vi "test Finalize Validation.vi"(8 "error in (no error)":errorcluster, 11 "TestCase in":refnum<class "Routing and Faulting Validation Unit Tests.lvclass">) -> (0 "error out":errorcluster, 3 "TestCase out":refnum<class "Routing and Faulting Validation Unit Tests.lvclass">)   [LabVIEW 2020, in "Routing and Faulting Validation Unit Tests.lvclass"]
uses:
  Routing and Faulting Validation Unit Tests.lvclass
  Routing and Faulting Validation Unit Tests.lvclass/Routing and Faulting Validation Unit Tests.ctl
  NationalInstruments.VeriStand.SystemStorage
  Constants/Scripting Constants.vi
  <vilib>/addons/_JKI Toolkits/VI Tester/TestCase.llb/TestCase.lvclass
  <vilib>/NI VeriStand/Custom Device API/Custom Device API.lvlib
  Routing and Faulting Scripting.lvlib
  C:/Program Files (x86)/National Instruments/LabVIEW 2020/vi.lib/addons/_JKI Toolkits/VI Tester/TestCase.llb/TestCase.lvclass
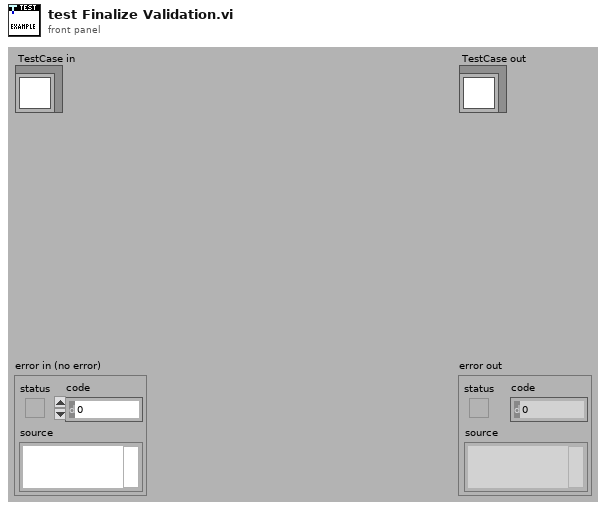
[diagram p1: front panel]
types:
  T1 = typedef "Custom Device API.lvlib/Custom Device Item Ref.ctl" = u64
  T2 = typedef "Routing and Faulting Scripting.lvlib/Validation Information.ctl" = cluster{"Missing Modules":variant, "Module Connection Map":variant, "Unused Modules":variant}
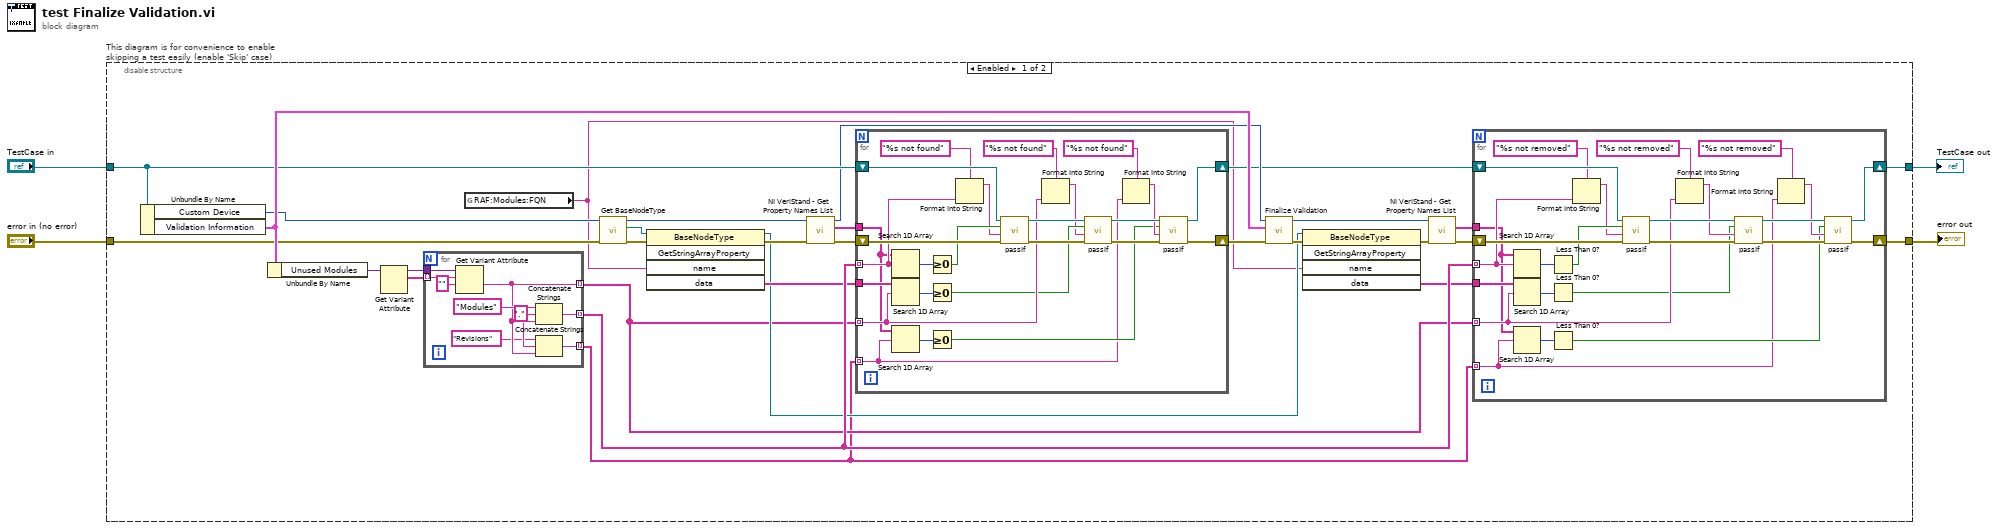
[diagram p0: block diagram]
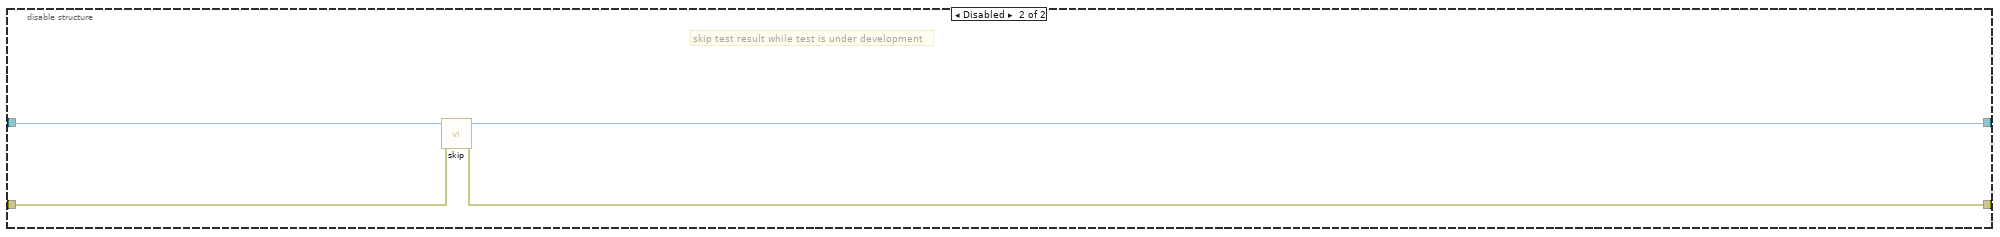
[diagram p2: hidden frame]
diagram:
  n1 = disable-structure "This diagram is for convenience to enable skipping a test easily (enable 'Skip' case)" shown="Enabled" {
    disable-tunnel: "TestCase in" -> [w29 w97]
    disable-tunnel: [w24 w95] -> w1
    disable-tunnel: [w23 w96] -> w3
    disable-tunnel: "error in (no error)" -> [w18 w94]
    frame Enabled {
      n2 = Unbundle By Name(w29) -> ("Custom Device"=w17:T1, "Validation Information"=w33:T2)
      n3 = Unbundle By Name(w33) -> ("Unused Modules"=w32:variant)
      n4 = Get Variant Attribute(Variant=w32) -> (duplicate Variant=w31:variant, names=w30:string[])  [unwired: 3 in, 2 out]
      n5 = for {
        tunnel: w31 -> [w93]
        tunnel: w30 -> [w92] mode=indexing
        tunnel: [w90] -> w19 mode=indexing
        tunnel: [w88] -> w6 mode=indexing
        tunnel: [w85] -> w5 mode=indexing
        w87 = "." ("string")
        n6 = Get Variant Attribute(Variant=w93, name=w92, default value (empty Variant)="") -> (value=w88:string)  [unwired: 1 in, 3 out]
        n7 = Concatenate Strings("Modules" ("string"), w87, w88) -> (w90:string)
        n8 = Concatenate Strings("Revisions" ("string"), w87, w88) -> (w85:string)
      }
      n9 = global read "Scripting Constants.vi" "RAF:Modules:FQN"() -> (w8:string)
      n10 = call "Get BaseNodeType.vi"("error in"=w18, "item in"=w17) -> ("error out"=w15:errorcluster, "BaseNodeType"=w14:refnum<k24>, "item out"=w16:T1)  [unwired: 7 in]
      n11 = invoke class="BaseNodeType" method="GetStringArrayProperty"(reference=w14, error in=w15, "name"=w8) -> (reference out=w9:refnum<k24>, error out=w13:errorcluster, "data"=w12:string[])  [unwired: 2 in, 2 out]
      n12 = call <vilib>:"NI VeriStand - Get Property Names List.vi"("error in (no error)"=w13, "Item Ref in"=w16) -> ("error out"=w28:errorcluster, "Property Names"=w27:string[], "Item Ref out"=w25:T1)  [unwired: 7 in]
      n13 = for {
        shift-right: [w66] -> w22
        shift-left: w29 -> [w81]
        shift-right: [w65] -> w26
        shift-left: w28 -> [w84]
        tunnel: w27 -> [w61]
        tunnel: w19 -> [w78] mode=indexing
        tunnel: w6 -> [w74] mode=indexing
        tunnel: w12 -> [w69]
        tunnel: w5 -> [w60] mode=indexing
        n14 = Search 1D Array(1D array=w61, element=w78) -> (index of element=w83:i32)  [unwired: 1 in]
        n15 = Search 1D Array(1D array=w69, element=w74) -> (index of element=w73:i32)  [unwired: 1 in]
        n16 = Search 1D Array(1D array=w61, element=w60) -> (index of element=w70:i32)  [unwired: 1 in]
        n17 = Greater Or Equal To 0?(x=w83) -> (x >= 0?=w82:bool)
        n18 = Greater Or Equal To 0?(x=w73) -> (x >= 0?=w72:bool)
        n19 = Greater Or Equal To 0?(x=w70) -> (x >= 0?=w62:bool)
        n20 = Format Into String(format string="%s not found" ("message (\"\")"), w78) -> (resulting string=w79:string)  [unwired: 2 in, 1 out]
        n21 = call-dynamic "passIf.vi"("error in (no error)"=w84, "message (\"\")"=w79, "pass"=w82, "TestCase in"=w81) -> ("error out"=w77:errorcluster, "TestCase out"=w76:refnum<class "Routing and Faulting Validation Unit Tests.lvclass">)  [unwired: 6 in]
        n22 = Format Into String(format string="%s not found" ("message (\"\")"), w74) -> (resulting string=w71:string)  [unwired: 2 in, 1 out]
        n23 = call-dynamic "passIf.vi"("error in (no error)"=w77, "message (\"\")"=w71, "pass"=w72, "TestCase in"=w76) -> ("error out"=w68:errorcluster, "TestCase out"=w67:refnum<class "Routing and Faulting Validation Unit Tests.lvclass">)  [unwired: 6 in]
        n24 = Format Into String(format string="%s not found" ("message (\"\")"), w60) -> (resulting string=w63:string)  [unwired: 2 in, 1 out]
        n25 = call-dynamic "passIf.vi"("error in (no error)"=w68, "message (\"\")"=w63, "pass"=w62, "TestCase in"=w67) -> ("error out"=w65:errorcluster, "TestCase out"=w66:refnum<class "Routing and Faulting Validation Unit Tests.lvclass">)  [unwired: 6 in]
      }
      n26 = call "Finalize Validation.vi"("error in"=w26, "validation information"=w33, "routing and faulting in"=w25) -> ("error out"=w10:errorcluster, "routing and faulting out"=w34:T1)  [unwired: 7 in]
      n27 = invoke class="BaseNodeType" method="GetStringArrayProperty"(reference=w9, error in=w10, "name"=w8) -> (error out=w11:errorcluster, "data"=w7:string[])  [unwired: 2 in, 3 out]
      n28 = call <vilib>:"NI VeriStand - Get Property Names List.vi"("error in (no error)"=w11, "Item Ref in"=w34) -> ("error out"=w21:errorcluster, "Property Names"=w20:string[])  [unwired: 7 in, 1 out]
      n29 = for {
        shift-right: [w39] -> w24
        shift-left: w22 -> [w56]
        shift-right: [w38] -> w23
        shift-left: w21 -> [w59]
        tunnel: w20 -> [w44]
        tunnel: w19 -> [w53] mode=indexing
        tunnel: w7 -> [w48]
        tunnel: w6 -> [w47] mode=indexing
        tunnel: w5 -> [w35] mode=indexing
        n30 = Search 1D Array(1D array=w44, element=w53) -> (index of element=w58:i32)  [unwired: 1 in]
        n31 = Search 1D Array(1D array=w48, element=w47) -> (index of element=w46:i32)  [unwired: 1 in]
        n32 = Search 1D Array(1D array=w44, element=w35) -> (index of element=w43:i32)  [unwired: 1 in]
        n33 = Less Than 0?(x=w58) -> (x < 0?=w57:bool)
        n34 = Less Than 0?(x=w46) -> (x < 0?=w45:bool)
        n35 = Less Than 0?(x=w43) -> (x < 0?=w36:bool)
        n36 = Format Into String(format string="%s not removed" ("message (\"\")"), w53) -> (resulting string=w55:string)  [unwired: 2 in, 1 out]
        n37 = call-dynamic "passIf.vi"("error in (no error)"=w59, "message (\"\")"=w55, "pass"=w57, "TestCase in"=w56) -> ("error out"=w51:errorcluster, "TestCase out"=w52:refnum<class "Routing and Faulting Validation Unit Tests.lvclass">)  [unwired: 6 in]
        n38 = Format Into String(format string="%s not removed" ("message (\"\")"), w47) -> (resulting string=w49:string)  [unwired: 2 in, 1 out]
        n39 = call-dynamic "passIf.vi"("error in (no error)"=w51, "message (\"\")"=w49, "pass"=w45, "TestCase in"=w52) -> ("error out"=w42:errorcluster, "TestCase out"=w41:refnum<class "Routing and Faulting Validation Unit Tests.lvclass">)  [unwired: 6 in]
        n40 = Format Into String(format string="%s not removed" ("message (\"\")"), w35) -> (resulting string=w37:string)  [unwired: 2 in, 1 out]
        n41 = call-dynamic "passIf.vi"("error in (no error)"=w42, "message (\"\")"=w37, "pass"=w36, "TestCase in"=w41) -> ("error out"=w38:errorcluster, "TestCase out"=w39:refnum<class "Routing and Faulting Validation Unit Tests.lvclass">)  [unwired: 6 in]
      }
    }
    frame Disabled {
      # "skip test result while test is under development"
      n42 = call <vilib>:"skip.vi"("error in (no error)"=w94, "TestCase in"=w97) -> ("error out"=w96:errorcluster, "TestCase out"=w95:refnum<class "Routing and Faulting Validation Unit Tests.lvclass">)  [unwired: 8 in]
    }
  }
  "error out" <- w3
  "TestCase out" <- w1
